vi "Manual Vi.vi"() -> ()   [LabVIEW 2015]
uses:
  IR/Control 1.ctl
  <vilib>/ni845x/ni845x.llb/ni845xControl.ctl
  <vilib>/MakerHub/LINX/Public/Peripherals/PWM/PWM Set Duty Cycle 1 Chan.vi
  <vilib>/MakerHub/LINX/Public/Peripherals/Digital/Digital Write 1 Chan.vi
  <vilib>/MakerHub/LINX/Public/Peripherals/Analog/Analog Read 1 Chan.vi
  <vilib>/MakerHub/LINX/Public/Peripherals/Analog/Analog Read N Chans.vi
  <vilib>/MakerHub/LINX/Public/Peripherals/Digital/Digital Write N Chans.vi
  <vilib>/MakerHub/LINX/Private/Local IO/LinxAnalogRead.vi
  <vilib>/MakerHub/LINX/Public/Utilities/Check Channel.vi
  <vilib>/MakerHub/LINX/Private/Local IO/LinxDigitalWrite.vi
  <vilib>/MakerHub/LINX/Public/Peripherals/PWM/PWM Set Duty Cycle N Chans.vi
  <vilib>/MakerHub/LINX/Private/Utilties/Generate Error.vi
  <vilib>/addons/control/pid/autopid.llb/PID Online Autotuning (Relay Feedback).vi
  <vilib>/addons/control/pid/pid.llb/PID Control Input Filter (DBL).vi
  <vilib>/addons/control/pid/NI_PID_pid.lvlib
  <vilib>/MakerHub/LINX/LMH-LINX.lvlib
  <vilib>/addons/control/pid/NI_PID_autopid.lvlib
  <instrlib>/Harvard Apparatus PHD Ultra Series/Harvard Apparatus PHD Ultra Series.lvlib
panel:
  out "LED already on? 5":bool
  out "LED already on? 4":bool
  out "LED already on? 3":bool
  out "LED already on? 2":bool
  out "LED already on? 1":bool
  in  "Flowrate":dbl=200.0
  in  "Pump Address":string="h"
  in  "LED On? 5":bool
  in  "LED On? 4":bool
  in  "LED On? 3":bool
  in  "LED On? 2":bool
  in  "LED On? 1":bool
  in  "HPLC with time(min)":dbl
  in  "Turn Valve and HPLC":bool
  in  "Turn HPLC":bool
  in  "Turn Valve":bool
  in  "Phase Sensor UB":dbl
  in  "Phase Sensor LB":dbl
  out "Pump On 7":bool=TRUE
  in  "Syringe Pump \n    Flowrate":dbl=200.0
  in  "Pump 7":bool
  out "Phase Sensor Chart":T1(graph)
  out "Phase_Sensor_voltage":dbl
  out "Temp SS 5":bool=TRUE
  out "Temp SS 4":bool=TRUE
  out "Temp SS 3":bool=TRUE
  out "Temp SS 2":bool=TRUE
  out "Temp SS 1":bool=TRUE
  in  "Temp On? 5":bool
  in  "Temp On? 4":bool
  in  "Temp On? 3":bool
  in  "Temp On? 2":bool
  in  "Temp On? 1":bool
  in  "Set Point 5":dbl
  in  "Set Point 4":dbl
  in  "Set Point 3":dbl
  in  "Set Point 2":dbl
  in  "Set Point 1":dbl
  in  "SSR Duration 5":dbl
  in  "SSR Duration 4":dbl
  in  "SSR Duration 3":dbl
  in  "SSR Duration 2":dbl
  in  "SSR Duration 1":dbl
  out "Pressure Chart 3":T1(graph)
  out "Flowrate Chart 3":T1(graph)
  out "System Error":bool=TRUE
  out "Flowrate Sensor 2":dbl format="%#_13g"
  out "Flowrate Sensor 1":dbl format="%#_13g"
  out "Pressure 2":dbl format="%#_13g"
  out "Pressure 1":dbl format="%#_13g"
  out "Error Message":string
  out "error out":errorcluster
  out "Temperature 4":dbl format="%#_g'C"
  out "Temperature 2":dbl format="%#_g'C"
  out "Temperature 5":dbl format="%#_g'C"
  out "Temperature 3":dbl format="%#_g'C"
  out "Temperature 1":dbl format="%#_g'C"
  out "Teperature Chart":T1(graph)
  out "Pump On 6":bool=TRUE
  out "Pump On 5":bool=TRUE
  out "Pump On 4":bool=TRUE
  out "Pump On 3":bool=TRUE
  out "Pump On 2":bool=TRUE
  out "Pump On 1":bool=TRUE
  in  "Stop Button":bool
  in  "Pump 6":bool
  in  "Pump 5":bool
  in  "Pump 4":bool
  in  "Pump 3":bool
  in  "Pump 2":bool
  in  "Pump 1":bool
  in  "Pump Address 6":string="h"
  in  "Pump Address 5":string="f"
  in  "Pump Address 4":string="e"
  in  "Pump Address 3":string="i"
  in  "Pump Address 2":string="j"
  in  "Pump Address 1":string="g"
  in  "Flowrate 6":dbl=200.0
  in  "Flowrate 5":dbl=200.0
  in  "Flowrate 4":dbl=200.0
  in  "Flowrate 3":dbl=200.0
  in  "Flowrate 2":dbl=200.0
  in  "Flowrate 1":dbl=200.0
  in  "COMM Port:: Harvard Syringe Pump":refnum<visa-resource-name>="COM5"
  in  "Sample Valve COMM::Port":refnum<visa-resource-name>="COM4"
  in  "IR Sensor Device":T2="USB0::0x3923::0x7514::01B3FF21::RAW"
  in  "Arduino COMM Port":refnum<visa-resource-name>="COM3"
  in  "COMM Port :: Milligat Pumps":T3="COM10"
  # "Molecules on Demand"
  # "Analytics"
  # "Pumps"
  # "Turn Valve and HPLC"
  # "Turn Valve"
  # "Turn on HPLC"
  # "Temperature Control"
  # "LED Reactors"
  # "Cooling Pump"
  # "Bay 2"
  # "Bay 3"
  # "Bay 1"
  # "Bay 4"
  # "Bay 5"
  # "Power On"
  # "Bay 1"
  # "Bay 2"
  # "Bay 3"
  # "Bay 4"
  # "Bay 5"
  # "Flowrates"
  # "Pressure"
  # "Temperature"
  # "Phase Sensor"
types:
  T1 = cluster{"[0]":dbl, "[1]":dbl, "[2]":dbl, "[3]":dbl, "[4]":dbl, "[5]":dbl, "[6]":dbl, "[7]":dbl, "[8]":dbl}
  T2 = typedef "ni845xControl.ctl" = refnum<k21>
  T3 = typedef "Control 1.ctl" = refnum<visa-resource-name>
  T4 = cluster{"Proportional gain Kc":dbl, "Integral time Ti (sec)":dbl, "Derivative time Ti (sec)":dbl}
  T5 = cluster{"type of controller":enum16{"P", "PI", "PID"}, "relay cycles":i32, "relay amplitude":dbl, "control specifications":enum16{"Fast", "Normal", "Slow"}, "PV noise level":dbl}
  T6 = typedef "LMH-LINX.lvlib/LINX Ref.ctl" = cluster{"IO":T7, "Interface":T8, "LINX Device Config":T9}
  T7 = typedef "LMH-LINX.lvlib/Platform.ctl" = enum16{"Remote", "Local"}
  T8 = typedef "LMH-LINX.lvlib/Interface.ctl" = enum16{"Serial", "TCP"}
  T9 = typedef "LMH-LINX.lvlib/Device.lvlib/LINX Device Config.ctl" = cluster{"Interface":T8, "COM Port":refnum<visa-resource-name>, "TCP Configuration":T10, "Device Family":u8, "Device ID":u8, "Device Name":string, "TCP Ref":refnum<k5>, "Channels":T11}
  T10 = typedef "LMH-LINX.lvlib/Device.lvlib/TCP Config.ctl" = cluster{"IP Address":string, "Port":u16}
  T11 = typedef "LMH-LINX.lvlib/Channels.ctl" = cluster{"DI":u8[], "DO":u8[], "AI":u8[], "AO":u8[], "PWM":u8[], "QE":u8[], "UART":u8[], "I2C 2":u8[], "SPI":u8[], "CAN":u8[], "Servo":u8[], "AI Ref (V)":dbl, "AI Resolution (Bits)":u8, "AO Ref (V)":dbl, "AO Resolution (Bits)":u8}
  T12 = cluster{"proportional gain (Kc)":dbl, "integral time (Ti, min)":dbl, "derivative time (Td, min)":dbl}
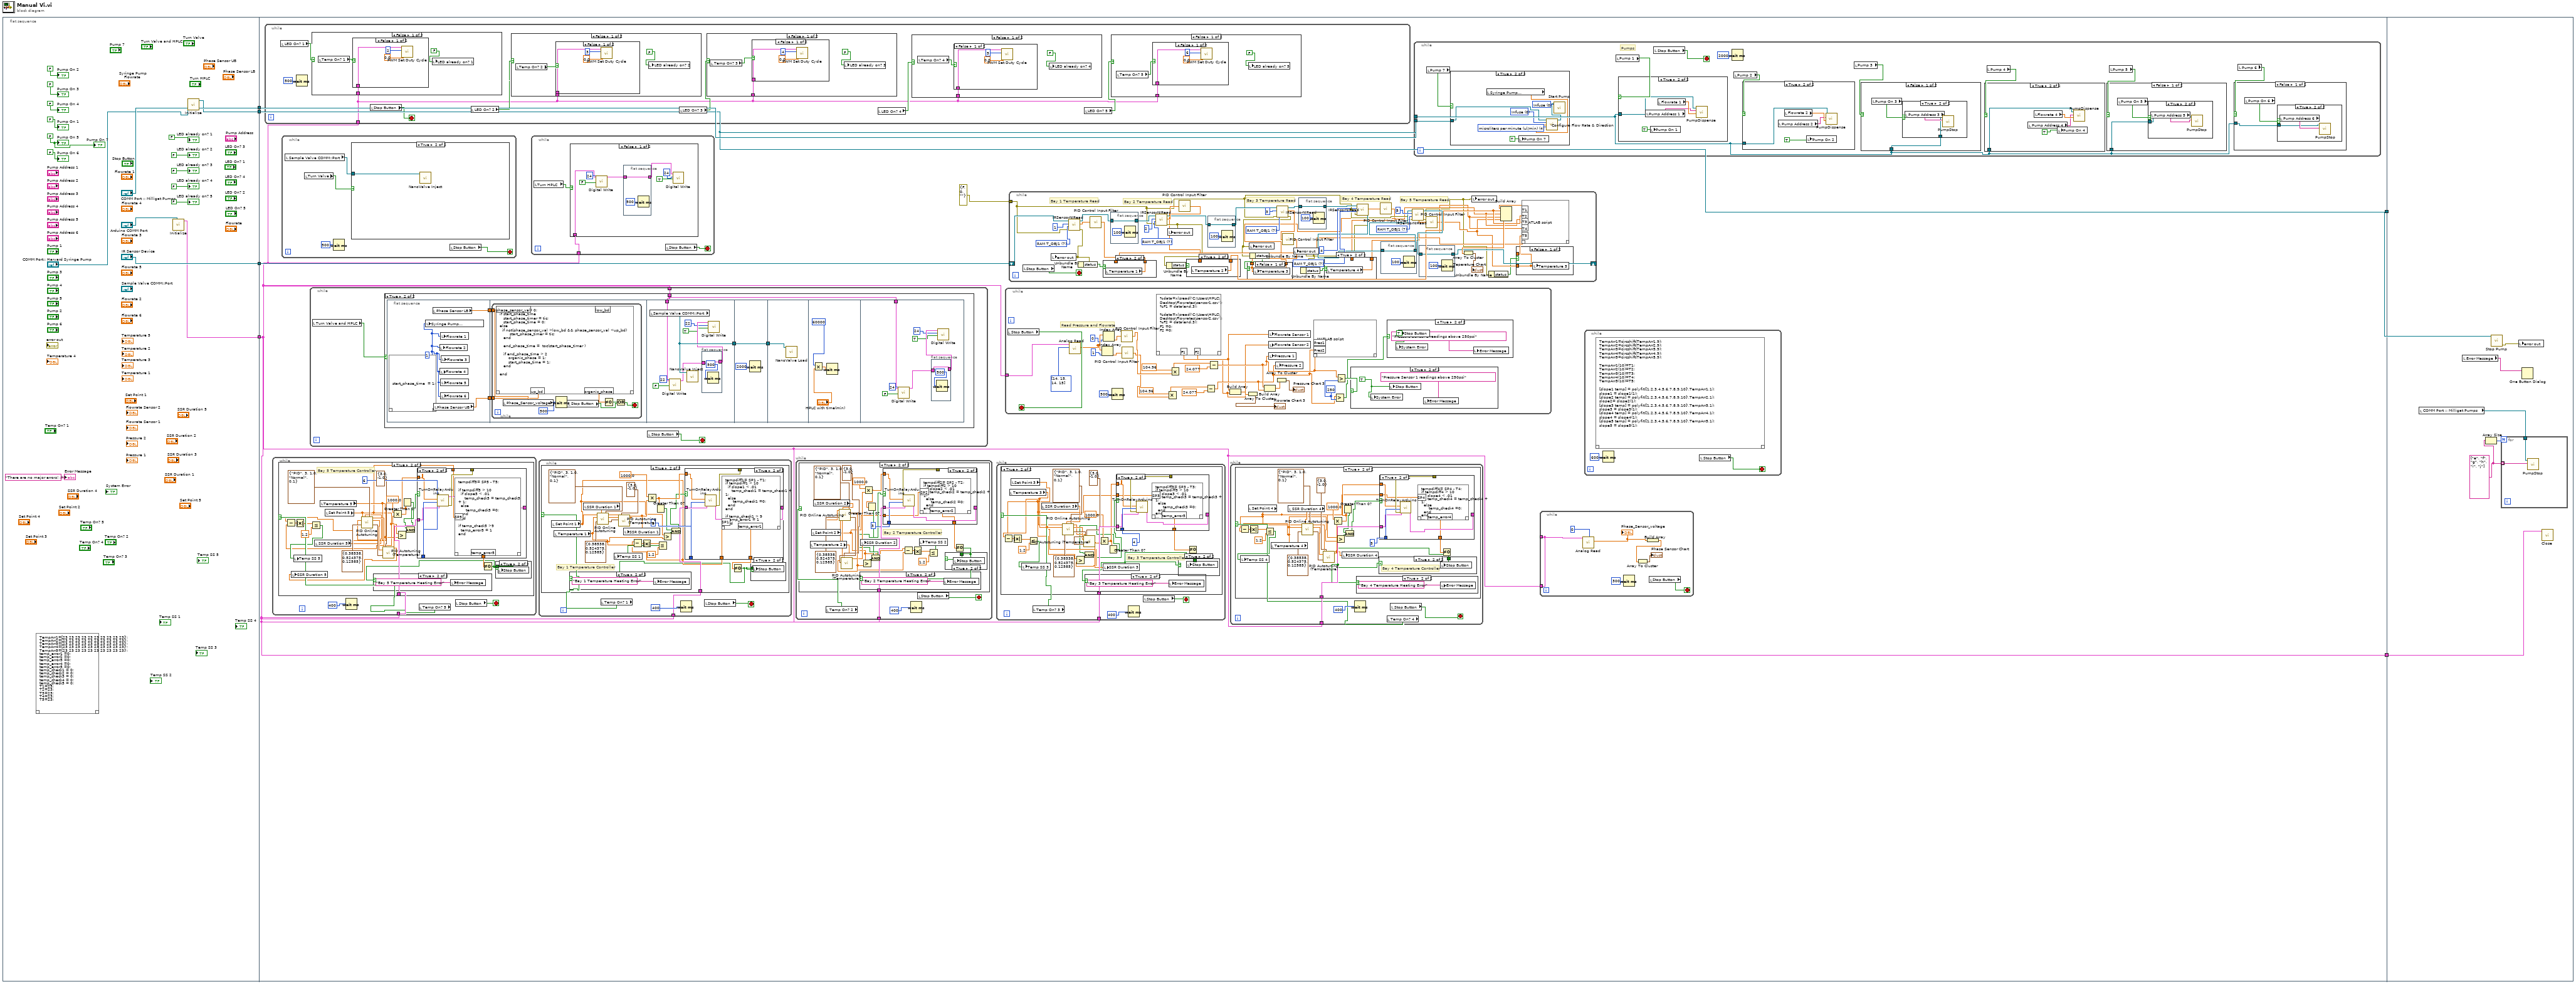
[diagram p0: block diagram]
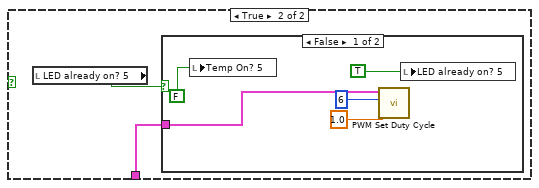
[diagram p3: hidden frame]
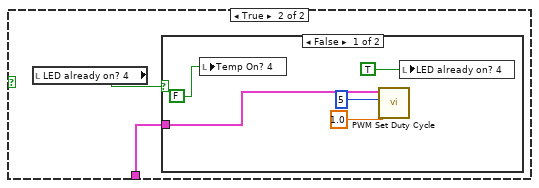
[diagram p6: hidden frame]
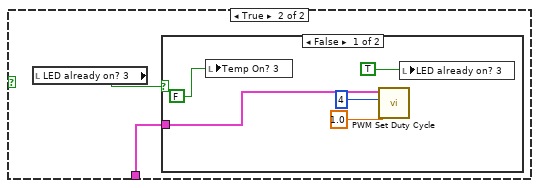
[diagram p9: hidden frame]
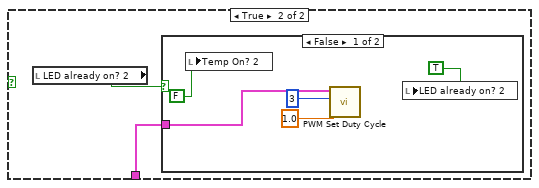
[diagram p12: hidden frame]
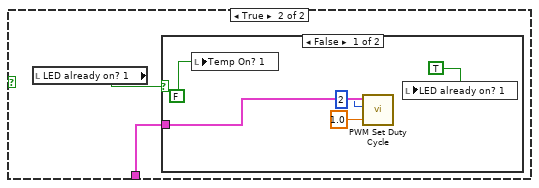
[diagram p15: hidden frame]
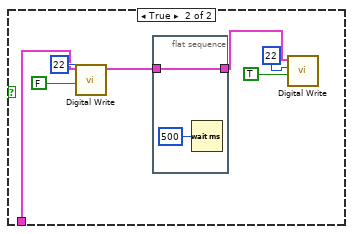
[diagram p18: hidden frame]
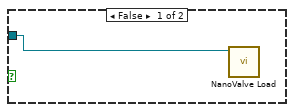
[diagram p19: hidden frame]
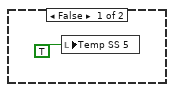
[diagram p20: hidden frame]
diagram:
  n1 = flat-sequence {
    tunnel: ["COMM Port :: Milligat Pumps"] -> w6
    tunnel: ["IR Sensor Device"] -> w5
    tunnel: [w16] -> w4
    tunnel: [w12] -> w2
    tunnel: w6 -> [w29]
    tunnel: w5 -> [w27]
    tunnel: w4 -> [w25]
    tunnel: [w25] -> w3
    tunnel: w2 -> [w26]
    tunnel: [w26] -> w1
    tunnel: w3 -> [w571]
    tunnel: w1 -> [w570]
    frame #0 {
      w14 = FALSE
      n2 = script code="TempArr1=[23 23 23 23 23 23 23 23 23 23]';\nTempArr2=[23 23 23 23 23 23 23 23 23 23]';\nTempArr3=[23 23 23 23 23 23 23 23 23 23]';\nTempArr4=[23 23 23 23 23 23 23 23 23 23]';\nTempArr5=[23 23 23 23 23 23 23 23 23 23]';\ntemp_error1 =0;\ntemp_error2 =0;\ntemp_error3 =0;\ntemp_error4 =0;\ntemp_error5 =0;\ntemp_check1 = 0;\ntemp_check2 = 0;\ntemp_check3 = 0;\ntemp_check4 = 0;\ntemp_check5 = 0;\nT1=23;\nT2=23;\nT3=23;\nT4=23;\nT5=23;"() -> ()  [unwired: 1 in, 1 out]
      n3 = call <instrlib>:"Initialize.vi"("Serial Port"="Arduino COMM Port") -> ("LINX Resource"=w16:T6)  [unwired: 8 in, 2 out]
      n4 = call <instrlib>:"Initialize.vi"("VISA resource name"="COMM Port:: Harvard Syringe Pump") -> ("VISA resource name out"=w12:refnum<visa-resource-name>)  [unwired: 9 in, 1 out]
      "Pump On 1" <- FALSE
      "Pump On 2" <- FALSE
      "Pump On 3" <- FALSE
      "Pump On 4" <- FALSE
      "Pump On 5" <- w14
      "Pump On 6" <- FALSE
      "Error Message" <- "There are no major errors! :)" ("Error Message")
      "Pump On 7" <- w14
      "LED already on? 1" <- FALSE ("LED already on? 1")
      "LED already on? 2" <- FALSE ("LED already on? 2")
      "LED already on? 3" <- FALSE ("LED already on? 3")
      "LED already on? 4" <- FALSE ("LED already on? 4")
      "LED already on? 5" <- FALSE ("LED already on? 5")
    }
    frame #1 {
      n5 = while {
        tunnel: w25 -> [w30]
        stop <- w37 stop-if-true
        n6 = local read "LED On? 1"() -> (w36:bool)
        n7 = Wait (ms)(milliseconds to wait=u32 500) -> ()  [unwired: 1 out]
        n8 = case shown="False" w36 {
          tunnel: w30 -> [w92 w96]
          frame False {
            n9 = local read "Temp On? 1"() -> (w90:bool)
            n10 = case shown="False" w90 {
              tunnel: w92 -> [w95 _]
              frame False {
                n11 = call-poly <vilib>:"PWM Set Duty Cycle.vi"("Duty Cycle (0-1)"=0.0, "PWM Channel"=u8 2, "LINX Resource"=w95) -> ()  [unwired: 7 in, 2 out]
              }
              frame True {
              }
            }
            n12 = local write "LED already on? 1"(FALSE ("LED already on? 2")) -> ()
          }
          frame True {
            n13 = local read "LED already on? 1"() -> (w97:bool)
            n14 = case shown="False" w97 {
              tunnel: w96 -> [w102 _]
              frame False {
                n15 = local write "Temp On? 1"(FALSE ("LED already on? 2")) -> ()
                n16 = call-poly <vilib>:"PWM Set Duty Cycle.vi"("Duty Cycle (0-1)"=1.0, "PWM Channel"=u8 2, "LINX Resource"=w102) -> ()  [unwired: 7 in, 2 out]
                n17 = local write "LED already on? 1"(TRUE ("LED already on? 2")) -> ()
              }
              frame True {
              }
            }
          }
        }
        n18 = local read "Stop Button"() -> (w37:bool)
        n19 = local read "LED On? 2"() -> (w34:bool)
        n20 = case shown="False" w34 {
          tunnel: w30 -> [w79 w83]
          frame False {
            n21 = local read "Temp On? 2"() -> (w77:bool)
            n22 = case shown="False" w77 {
              tunnel: w79 -> [w82 _]
              frame False {
                n23 = call-poly <vilib>:"PWM Set Duty Cycle.vi"("Duty Cycle (0-1)"=0.0, "PWM Channel"=u8 3, "LINX Resource"=w82) -> ()  [unwired: 7 in, 2 out]
              }
              frame True {
              }
            }
            n24 = local write "LED already on? 2"(FALSE ("LED already on? 2")) -> ()
          }
          frame True {
            n25 = local read "LED already on? 2"() -> (w84:bool)
            n26 = case shown="False" w84 {
              tunnel: w83 -> [w89 _]
              frame False {
                n27 = local write "Temp On? 2"(FALSE ("LED already on? 2")) -> ()
                n28 = call-poly <vilib>:"PWM Set Duty Cycle.vi"("Duty Cycle (0-1)"=1.0, "PWM Channel"=u8 3, "LINX Resource"=w89) -> ()  [unwired: 7 in, 2 out]
                n29 = local write "LED already on? 2"(TRUE ("LED already on? 2")) -> ()
              }
              frame True {
              }
            }
          }
        }
        n30 = local read "LED On? 3"() -> (w33:bool)
        n31 = case shown="False" w33 {
          tunnel: w30 -> [w66 w70]
          frame False {
            n32 = local read "Temp On? 3"() -> (w64:bool)
            n33 = case shown="False" w64 {
              tunnel: w66 -> [w69 _]
              frame False {
                n34 = call-poly <vilib>:"PWM Set Duty Cycle.vi"("Duty Cycle (0-1)"=0.0, "PWM Channel"=u8 4, "LINX Resource"=w69) -> ()  [unwired: 7 in, 2 out]
              }
              frame True {
              }
            }
            n35 = local write "LED already on? 3"(FALSE ("LED already on? 2")) -> ()
          }
          frame True {
            n36 = local read "LED already on? 3"() -> (w71:bool)
            n37 = case shown="False" w71 {
              tunnel: w70 -> [w76 _]
              frame False {
                n38 = local write "Temp On? 3"(FALSE ("LED already on? 2")) -> ()
                n39 = call-poly <vilib>:"PWM Set Duty Cycle.vi"("Duty Cycle (0-1)"=1.0, "PWM Channel"=u8 4, "LINX Resource"=w76) -> ()  [unwired: 7 in, 2 out]
                n40 = local write "LED already on? 3"(TRUE ("LED already on? 2")) -> ()
              }
              frame True {
              }
            }
          }
        }
        n41 = local read "LED On? 4"() -> (w32:bool)
        n42 = case shown="False" w32 {
          tunnel: w30 -> [w53 w57]
          frame False {
            n43 = local read "Temp On? 4"() -> (w51:bool)
            n44 = case shown="False" w51 {
              tunnel: w53 -> [w56 _]
              frame False {
                n45 = call-poly <vilib>:"PWM Set Duty Cycle.vi"("Duty Cycle (0-1)"=0.0, "PWM Channel"=u8 5, "LINX Resource"=w56) -> ()  [unwired: 7 in, 2 out]
              }
              frame True {
              }
            }
            n46 = local write "LED already on? 4"(FALSE ("LED already on? 2")) -> ()
          }
          frame True {
            n47 = local read "LED already on? 4"() -> (w58:bool)
            n48 = case shown="False" w58 {
              tunnel: w57 -> [w63 _]
              frame False {
                n49 = local write "Temp On? 4"(FALSE ("LED already on? 2")) -> ()
                n50 = call-poly <vilib>:"PWM Set Duty Cycle.vi"("Duty Cycle (0-1)"=1.0, "PWM Channel"=u8 5, "LINX Resource"=w63) -> ()  [unwired: 7 in, 2 out]
                n51 = local write "LED already on? 4"(TRUE ("LED already on? 2")) -> ()
              }
              frame True {
              }
            }
          }
        }
        n52 = local read "LED On? 5"() -> (w31:bool)
        n53 = case shown="False" w31 {
          tunnel: w30 -> [w40 w44]
          frame False {
            n54 = local read "Temp On? 5"() -> (w38:bool)
            n55 = case shown="False" w38 {
              tunnel: w40 -> [w43 _]
              frame False {
                n56 = call-poly <vilib>:"PWM Set Duty Cycle.vi"("Duty Cycle (0-1)"=0.0, "PWM Channel"=u8 6, "LINX Resource"=w43) -> ()  [unwired: 7 in, 2 out]
              }
              frame True {
              }
            }
            n57 = local write "LED already on? 5"(FALSE ("LED already on? 2")) -> ()
          }
          frame True {
            n58 = local read "LED already on? 5"() -> (w45:bool)
            n59 = case shown="False" w45 {
              tunnel: w44 -> [w50 _]
              frame False {
                n60 = local write "Temp On? 5"(FALSE ("LED already on? 2")) -> ()
                n61 = call-poly <vilib>:"PWM Set Duty Cycle.vi"("Duty Cycle (0-1)"=1.0, "PWM Channel"=u8 6, "LINX Resource"=w50) -> ()  [unwired: 7 in, 2 out]
                n62 = local write "LED already on? 5"(TRUE ("LED already on? 2")) -> ()
              }
              frame True {
              }
            }
          }
        }
      }
      n63 = while {
        tunnel: w25 -> [w187]
        stop <- w186 stop-if-true
        n64 = Wait (ms)(milliseconds to wait=u32 400) -> ()  [unwired: 1 out]
        n65 = local read "Temp On? 5"() -> (w185:bool)
        n66 = case shown="True" w185 {
          tunnel: w187 -> [_ w211]
          frame False {
            n67 = local write "Temp SS 5"(TRUE ("Temp SS? 5")) -> ()
          }
          frame True {
            # "Bay 5 Temperature Controller"
            n68 = local read "SSR Duration 5"() -> (w201:dbl)
            n69 = local read "Temperature 5"() -> (w193:dbl)
            n70 = local read "Set Point 5"() -> (w191:dbl)
            n71 = Subtract(x=w193, y=w191) -> (x-y=w198:dbl)
            n72 = Absolute Value(x=w198) -> (abs(x)=w200:dbl)
            n73 = Less Or Equal?(x=w200, y=1.2) -> (x <= y?=w197:bool)
            n74 = local write "Temp SS 5"(w197) -> ()
            n75 = call-poly <vilib>:"PID Online Autotuning.vi"("setpoint"=w191, "manipulated variable"=w201, "autotuning parameters"=T5 {"type of controller"=enum."PID", "relay cycles"=3, "relay amplitude"=1.0, "control specifications"=enum."Normal", "PV noise level"=0.1} ("Autotuning Parameters R1"), "process variable"=w193, "PID gains in"=T4 {"Proportional gain Kc"=0.38538, "Integral time Ti (sec)"=0.524375, "Derivative time Ti (sec)"=0.12585} ("PID gains 2")) -> ("setpoint out"=w203:dbl, "process variable out"=w204:dbl, "PID gains out"=w206:T12)  [unwired: 6 in, 2 out]
            n76 = call <vilib>:"PID Autotuning (Temperature).vi"("desired temperature"=w203, "measured temperature"=w204, "PID gains in"=w206, "output range"=cluster{"output high":dbl, "output low":dbl} {"output high"=3.0, "output low"=-1.0} ("Output range")) -> ("output"=w202:dbl)  [unwired: 12 in, 3 out]
            n77 = local write "SSR Duration 5"(w202) -> ()
            n78 = Multiply(x=1000.0, y=w202) -> (x*y=w210:dbl)
            n79 = Greater?(x=w191, y=w193) -> (0:w194:bool)
            n80 = Greater Than 0?(x=w210) -> (x > 0?=w196:bool)
            n81 = And(x=w196, y=w194) -> (x .and. y?=w195:bool)
            n82 = case shown="True" w195 {
              tunnel: [errorcluster {"status"=FALSE, "code"=0, "source"=""} ("error out") w225] -> _
              tunnel: 6 -> [_ w226]
              tunnel: [w217 w224] -> _
              tunnel: w211 -> [w217 w223]
              tunnel: w210 -> [w216 w222]
              tunnel: [0.0 w221] -> w192
              tunnel: w191 -> [_ w220]
              frame False {
                n83 = Absolute Value(x=w216) -> (abs(x)=w218:dbl)
                n84 = Wait (ms)(milliseconds to wait=w218) -> ()  [unwired: 1 out]
              }
              frame True {
                n85 = call "TurnOnRelayArduino.vi"("channel"=w226, "duration"=w222, "LINX Resource"=w223) -> ("error out"=w225:errorcluster, "LINX Resource Out"=w224:T6)  [unwired: 7 in]
                n86 = script code="tempdiff5= SP5 - T5;\n\nif tempdiff5 > 10\n  if slope5 < .01\n     temp_check5 = temp_check5 + 1;\n  else\n      temp_check5 =0;\n  end\nend\n\nif temp_check5 >9\n  temp_error5 = 1\nend"("SP5"=w220) -> ("temp_error5"=w221:dbl)  [unwired: 1 in, 1 out]
              }
            }
            n87 = Not Equal To 0?(x=w192) -> (x != 0?=w190:bool)
            n88 = case shown="True" w190 {
              frame False {
              }
              frame True {
                n89 = local write "Error Message"("Bay 5 Temperature Heating Error") -> ()
              }
            }
            n90 = case shown="True" w190 {
              tunnel: w190 -> [_ w213]
              frame False {
              }
              frame True {
                n91 = local write "Stop Button"(w213) -> ()
              }
            }
          }
        }
        n92 = local read "Stop Button"() -> (w186:bool)
      }
      n93 = while {
        stop <- w175 stop-if-true
        n94 = local read "Sample Valve COMM::Port"() -> (w172:refnum<visa-resource-name>)
        n95 = local read "Turn Valve"() -> (w173:bool)
        n96 = Wait (ms)(milliseconds to wait=u32 500) -> ()  [unwired: 1 out]
        n97 = case shown="True" w173 {
          tunnel: w172 -> [w176 w177]
          frame False {
            n98 = call "NanoValve Load.vi"("VISA resource name"=w176) -> ()  [unwired: 10 in, 1 out]
          }
          frame True {
            n99 = call "NanoValve Inject.vi"("VISA resource name"=w177) -> ()  [unwired: 10 in, 1 out]
          }
        }
        n100 = local read "Stop Button"() -> (w175:bool)
      }
      n101 = while {
        tunnel: w25 -> [w105]
        stop <- w107 stop-if-true
        n102 = local read "Turn Valve and HPLC"() -> (w106:bool)
        n103 = case shown="True" w106 {
          tunnel: w105 -> [_ w108]
          frame False {
          }
          frame True {
            n104 = flat-sequence {
              tunnel: [w114] -> w110
              tunnel: [w113] -> w109
              tunnel: w110 -> [w117]
              tunnel: w109 -> [w116]
              tunnel: w108 -> [w131]
              tunnel: [w130] -> w111
              tunnel: [w136] -> w112
              tunnel: w111 -> [w136]
              tunnel: w112 -> [w138]
              tunnel: w108 -> [w142]
              frame #0 {
                w115 = 1
                n105 = script code="start_phase_time  = 1;"() -> ()  [unwired: 1 in, 1 out]
                n106 = local write "Syringe Pump \n    Flowrate"(w115) -> ()
                n107 = local read "Phase Sensor LB"() -> (w113:dbl)
                n108 = local read "Phase Sensor UB"() -> (w114:dbl)
                n109 = local write "Flowrate 2"(w115) -> ()
                n110 = local write "Flowrate 4"(w115) -> ()
                n111 = local write "Flowrate 1"(w115) -> ()
                n112 = local write "Flowrate 5"(w115) -> ()
                n113 = local write "Flowrate 6"(w115) -> ()
                n114 = local write "Flowrate 3"(w115) -> ()
              }
              frame #1 {
                n115 = while {
                  tunnel: w117 -> [w119]
                  tunnel: w116 -> [w118]
                  stop <- w122 stop-if-true
                  n116 = local read "Phase_Sensor_voltage"() -> (w125:dbl)
                  n117 = script code="organic_phase = 0;\nif start_phase_time \n   start_phase_timer = tic;\n   start_phase_time = 0;\nelse\n  if not(phase_sensor_val >low_bd && phase_sensor_val <up_bd)\n        start_phase_timer = tic;\n   end\n\n   end_phase_time =  toc(start_phase_timer )\n\n   if end_phase_time > 2\n       organic_phase = 1;\n       start_phase_time = 1;\n   end\n\nend"("phase_sensor_val"=w125, "low_bd"=w118, "up_bd"=w119) -> ("organic_phase"=w124:dbl)  [unwired: 1 in, 1 out]
                  n118 = Wait (ms)(milliseconds to wait=500) -> ()  [unwired: 1 out]
                  n119 = local read "Stop Button"() -> (w121:bool)
                  n120 = Not Equal To 0?(x=w124) -> (x != 0?=w123:bool)
                  n121 = Or(x=w123, y=w121) -> (x .or. y?=w122:bool)
                }
              }
              frame #2 {
                n122 = local read "Sample Valve COMM::Port"() -> (w130:refnum<visa-resource-name>)
                n123 = call-poly <vilib>:"Digital Write.vi"("Output Value"=FALSE, "DO Channel"=u8 22, "LINX Resource"=w131) -> ("LINX Resource"=w129:T6)  [unwired: 7 in, 1 out]
                n124 = call "NanoValve Inject.vi"("VISA resource name"=w130) -> ()  [unwired: 10 in, 1 out]
                n125 = flat-sequence {
                  tunnel: [w134] -> _
                  tunnel: w129 -> [w134]
                  tunnel: [w134] -> w128
                  frame #0 {
                    n126 = Wait (ms)(milliseconds to wait=u32 500) -> ()  [unwired: 1 out]
                  }
                }
                n127 = call-poly <vilib>:"Digital Write.vi"("Output Value"=TRUE, "DO Channel"=u8 22, "LINX Resource"=w128) -> ()  [unwired: 7 in, 2 out]
              }
              frame #3 {
                n128 = Wait (ms)(milliseconds to wait=u32 2000) -> ()  [unwired: 1 out]
              }
              frame #4 {
                n129 = call "NanoValve Load.vi"("VISA resource name"=w138) -> ()  [unwired: 10 in, 1 out]
              }
              frame #5 {
                n130 = Multiply(x=u32 60000 ("milliseconds to wait"), y="HPLC with time(min)") -> (x*y=w140:dbl)
                n131 = Wait (ms)(milliseconds to wait=w140) -> ()  [unwired: 1 out]
              }
              frame #6 {
                n132 = call-poly <vilib>:"Digital Write.vi"("Output Value"=FALSE, "DO Channel"=u8 24, "LINX Resource"=w142) -> ("LINX Resource"=w146:T6)  [unwired: 7 in, 1 out]
                n133 = flat-sequence {
                  tunnel: w146 -> [w149]
                  tunnel: [w149] -> w145
                  frame #0 {
                    n134 = Wait (ms)(milliseconds to wait=u32 500) -> ()  [unwired: 1 out]
                  }
                }
                n135 = call-poly <vilib>:"Digital Write.vi"("Output Value"=TRUE, "DO Channel"=u8 24, "LINX Resource"=w145) -> ()  [unwired: 7 in, 2 out]
              }
            }
          }
        }
        n136 = local read "Stop Button"() -> (w107:bool)
      }
      n137 = while {
        tunnel: w25 -> [w151]
        stop <- w153 stop-if-true
        n138 = local read "Turn HPLC"() -> (w152:bool)
        n139 = case shown="False" w152 {
          tunnel: w151 -> [w154 w167]
          frame False {
            n140 = call-poly <vilib>:"Digital Write.vi"("Output Value"=FALSE, "DO Channel"=u8 24, "LINX Resource"=w154) -> ("LINX Resource"=w158:T6)  [unwired: 7 in, 1 out]
            n141 = flat-sequence {
              tunnel: [w161] -> w155
              tunnel: w158 -> [w161]
              frame #0 {
                n142 = Wait (ms)(milliseconds to wait=u32 500) -> ()  [unwired: 1 out]
              }
            }
            n143 = call-poly <vilib>:"Digital Write.vi"("Output Value"=TRUE, "DO Channel"=u8 24, "LINX Resource"=w155) -> ()  [unwired: 7 in, 2 out]
          }
          frame True {
            n144 = call-poly <vilib>:"Digital Write.vi"("Output Value"=FALSE, "DO Channel"=u8 22, "LINX Resource"=w167) -> ("LINX Resource"=w166:T6)  [unwired: 7 in, 1 out]
            n145 = flat-sequence {
              tunnel: [w170] -> w163
              tunnel: w166 -> [w170]
              frame #0 {
                n146 = Wait (ms)(milliseconds to wait=u32 500) -> ()  [unwired: 1 out]
              }
            }
            n147 = call-poly <vilib>:"Digital Write.vi"("Output Value"=TRUE, "DO Channel"=u8 22, "LINX Resource"=w163) -> ()  [unwired: 7 in, 2 out]
          }
        }
        n148 = local read "Stop Button"() -> (w153:bool)
      }
      n149 = while {
        tunnel: w25 -> [w354]
        stop <- w356 stop-if-true
        n150 = local read "Temp On? 1"() -> (w353:bool)
        n151 = case shown="True" w353 {
          tunnel: w354 -> [_ w370]
          frame False {
            n152 = local write "Temp SS 1"(TRUE ("Temp SS? 1")) -> ()
          }
          frame True {
            # "Bay 1 Temperature Controller"
            n153 = local read "Set Point 1"() -> (w359:dbl)
            n154 = local read "Temperature 1"() -> (w361:dbl)
            n155 = local read "SSR Duration 1"() -> (w374:dbl)
            n156 = call-poly <vilib>:"PID Online Autotuning.vi"("setpoint"=w359, "manipulated variable"=w374, "autotuning parameters"=T5 {"type of controller"=enum."PID", "relay cycles"=3, "relay amplitude"=1.0, "control specifications"=enum."Normal", "PV noise level"=0.1} ("Autotuning Parameters R1"), "process variable"=w361, "PID gains in"=T4 {"Proportional gain Kc"=0.38538, "Integral time Ti (sec)"=0.524375, "Derivative time Ti (sec)"=0.12585} ("PID gains 2")) -> ("setpoint out"=w380:dbl, "process variable out"=w379:dbl, "PID gains out"=w376:T12)  [unwired: 6 in, 2 out]
            n157 = call <vilib>:"PID Autotuning (Temperature).vi"("desired temperature"=w380, "measured temperature"=w379, "plant parameters in"=w376, "output range"=cluster{"output high":dbl, "output low":dbl} {"output high"=3.0, "output low"=-1.0} ("Output range")) -> ("output"=w372:dbl)  [unwired: 12 in, 3 out]
            n158 = local write "SSR Duration 1"(w372) -> ()
            n159 = Subtract(x=w359, y=w361) -> (x-y=w365:dbl)
            n160 = Absolute Value(x=w365) -> (abs(x)=w368:dbl)
            n161 = Multiply(x=1000.0, y=w372) -> (x*y=w369:dbl)
            n162 = Greater Than 0?(x=w369) -> (x > 0?=w362:bool)
            n163 = Less Or Equal?(x=w368, y=1.2) -> (x <= y?=w366:bool)
            n164 = local write "Temp SS 1"(w366) -> ()
            n165 = Greater?(x=w359, y=w361) -> (0:w364:bool)
            n166 = And(x=w362, y=w364) -> (x .and. y?=w363:bool)
            n167 = case shown="True" w363 {
              tunnel: [errorcluster {"status"=FALSE, "code"=0, "source"=""} ("error out") w392] -> _
              tunnel: w370 -> [w385 w394]
              tunnel: 2 -> [_ w393]
              tunnel: [w385 w391] -> _
              tunnel: w369 -> [w384 w390]
              tunnel: [0.0 w389] -> w360
              tunnel: w359 -> [_ w388]
              frame False {
                n168 = Absolute Value(x=w384) -> (abs(x)=w386:dbl)
                n169 = Wait (ms)(milliseconds to wait=w386) -> ()  [unwired: 1 out]
              }
              frame True {
                n170 = call "TurnOnRelayArduino.vi"("channel"=w393, "duration"=w390, "LINX Resource"=w394) -> ("error out"=w392:errorcluster, "LINX Resource Out"=w391:T6)  [unwired: 7 in]
                n171 = script code="tempdiff1= SP1 - T1;\nif tempdiff1 > 10\n  if slope1 < .01\n     temp_check1 = temp_check1 + 1;\n  else\n      temp_check1 =0;\n  end\nend\n\nif temp_check1 > 9\n  temp_error1 = 1\nend"("SP1"=w388) -> ("temp_error1"=w389:dbl)  [unwired: 1 in, 1 out]
              }
            }
            n172 = Not Equal To 0?(x=w360) -> (x != 0?=w358:bool)
            n173 = case shown="True" w358 {
              frame False {
              }
              frame True {
                n174 = local write "Error Message"("Bay 1 Temperature Heating Error") -> ()
              }
            }
            n175 = case shown="True" w358 {
              tunnel: w358 -> [_ w381]
              frame False {
              }
              frame True {
                n176 = local write "Stop Button"(w381) -> ()
              }
            }
          }
        }
        n177 = Wait (ms)(milliseconds to wait=u32 400) -> ()  [unwired: 1 out]
        n178 = local read "Stop Button"() -> (w356:bool)
      }
      n179 = while {
        tunnel: w25 -> [w312]
        stop <- w314 stop-if-true
        n180 = local read "Temp On? 2"() -> (w311:bool)
        n181 = case shown="True" w311 {
          tunnel: w312 -> [_ w331]
          frame False {
            n182 = local write "Temp SS 2"(TRUE ("Temp SS? 2")) -> ()
          }
          frame True {
            # "Bay 2 Temperature Controller"
            n183 = local read "Temperature 2"() -> (w319:dbl)
            n184 = local read "Set Point 2"() -> (w317:dbl)
            n185 = local read "SSR Duration 2"() -> (w335:dbl)
            n186 = call-poly <vilib>:"PID Online Autotuning.vi"("setpoint"=w317, "manipulated variable"=w335, "autotuning parameters"=T5 {"type of controller"=enum."PID", "relay cycles"=3, "relay amplitude"=1.0, "control specifications"=enum."Normal", "PV noise level"=0.1} ("Autotuning Parameters R1"), "process variable"=w319, "PID gains in"=T4 {"Proportional gain Kc"=0.38538, "Integral time Ti (sec)"=0.524375, "Derivative time Ti (sec)"=0.12585} ("PID gains 2")) -> ("setpoint out"=w333:dbl, "process variable out"=w332:dbl, "PID gains out"=w338:T12)  [unwired: 6 in, 2 out]
            n187 = call <vilib>:"PID Autotuning (Temperature).vi"("desired temperature"=w333, "measured temperature"=w332, "plant parameters in"=w338, "output range"=cluster{"output high":dbl, "output low":dbl} {"output high"=3.0, "output low"=-1.0} ("Output range")) -> ("output"=w327:dbl)  [unwired: 12 in, 3 out]
            n188 = local write "SSR Duration 2"(w327) -> ()
            n189 = Greater?(x=w317, y=w319) -> (0:w322:bool)
            n190 = Multiply(x=1000.0, y=w327) -> (x*y=w329:dbl)
            n191 = Greater Than 0?(x=w329) -> (x > 0?=w320:bool)
            n192 = And(x=w320, y=w322) -> (x .and. y?=w321:bool)
            n193 = case shown="True" w321 {
              tunnel: [errorcluster {"status"=FALSE, "code"=0, "source"=""} ("error out") w350] -> _
              tunnel: w331 -> [w343 w352]
              tunnel: 3 -> [_ w351]
              tunnel: [w343 w349] -> _
              tunnel: w329 -> [w342 w348]
              tunnel: [0.0 w347] -> w318
              tunnel: w317 -> [_ w346]
              frame False {
                n194 = Absolute Value(x=w342) -> (abs(x)=w344:dbl)
                n195 = Wait (ms)(milliseconds to wait=w344) -> ()  [unwired: 1 out]
              }
              frame True {
                n196 = call "TurnOnRelayArduino.vi"("channel"=w351, "duration"=w348, "LINX Resource"=w352) -> ("error out"=w350:errorcluster, "LINX Resource Out"=w349:T6)  [unwired: 7 in]
                n197 = script code="tempdiff2= SP2 - T2;\nif tempdiff2 > 10\n  if slope2 < .01\n     temp_check2 = temp_check2 + 1;\n  else\n      temp_check2 =0;\n  end\nend\n\nif temp_check2 > 9\n  temp_error2 = 1\nend"("SP2"=w346) -> ("temp_error2"=w347:dbl)  [unwired: 1 in, 1 out]
              }
            }
            n198 = Subtract(x=w317, y=w319) -> (x-y=w324:dbl)
            n199 = Absolute Value(x=w324) -> (abs(x)=w326:dbl)
            n200 = Less Or Equal?(x=w326, y=1.2) -> (x <= y?=w323:bool)
            n201 = local write "Temp SS 2"(w323) -> ()
            n202 = Not Equal To 0?(x=w318) -> (x != 0?=w316:bool)
            n203 = case shown="True" w316 {
              frame False {
              }
              frame True {
                n204 = local write "Error Message"("Bay 2 Temperature Heating Error") -> ()
              }
            }
            n205 = case shown="True" w316 {
              tunnel: w316 -> [_ w339]
              frame False {
              }
              frame True {
                n206 = local write "Stop Button"(w339) -> ()
              }
            }
          }
        }
        n207 = Wait (ms)(milliseconds to wait=u32 400) -> ()  [unwired: 1 out]
        n208 = local read "Stop Button"() -> (w314:bool)
      }
      n209 = while {
        tunnel: w25 -> [w270]
        stop <- w271 stop-if-true
        n210 = local read "Temp On? 3"() -> (w269:bool)
        n211 = case shown="True" w269 {
          tunnel: w270 -> [_ w296]
          frame False {
            n212 = local write "Temp SS 3"(TRUE) -> ()
          }
          frame True {
            # "Bay 3 Temperature Controller"
            n213 = local read "Temperature 3"() -> (w279:dbl)
            n214 = local read "Set Point 3"() -> (w275:dbl)
            n215 = Subtract(x=w279, y=w275) -> (x-y=w282:dbl)
            n216 = Absolute Value(x=w282) -> (abs(x)=w284:dbl)
            n217 = Less Or Equal?(x=w284, y=1.2) -> (x <= y?=w281:bool)
            n218 = local write "Temp SS 3"(w281) -> ()
            n219 = local read "SSR Duration 3"() -> (w291:dbl)
            n220 = call-poly <vilib>:"PID Online Autotuning.vi"("setpoint"=w275, "manipulated variable"=w291, "autotuning parameters"=T5 {"type of controller"=enum."PID", "relay cycles"=3, "relay amplitude"=1.0, "control specifications"=enum."Normal", "PV noise level"=0.1} ("Autotuning Parameters R1"), "process variable"=w279, "PID gains in"=T4 {"Proportional gain Kc"=0.38538, "Integral time Ti (sec)"=0.524375, "Derivative time Ti (sec)"=0.12585} ("PID gains 2")) -> ("setpoint out"=w289:dbl, "process variable out"=w290:dbl, "PID gains out"=w293:T12)  [unwired: 6 in, 2 out]
            n221 = Greater?(x=w275, y=w279) -> (0:w280:bool)
            n222 = call <vilib>:"PID Autotuning (Temperature).vi"("desired temperature"=w289, "measured temperature"=w290, "PID gains in"=w293, "output range"=cluster{"output high":dbl, "output low":dbl} {"output high"=3.0, "output low"=-1.0} ("Output range")) -> ("output"=w286:dbl)  [unwired: 12 in, 3 out]
            n223 = Multiply(x=1000.0, y=w286) -> (x*y=w288:dbl)
            n224 = local write "SSR Duration 3"(w286) -> ()
            n225 = Greater Than 0?(x=w288) -> (x > 0?=w278:bool)
            n226 = And(x=w278, y=w280) -> (x .and. y?=w277:bool)
            n227 = case shown="True" w277 {
              tunnel: [errorcluster {"status"=FALSE, "code"=0, "source"=""} ("error out") w309] -> _
              tunnel: 4 -> [_ w310]
              tunnel: [w301 w308] -> _
              tunnel: w296 -> [w301 w307]
              tunnel: w288 -> [w300 w306]
              tunnel: [0.0 w305] -> w276
              tunnel: w275 -> [_ w304]
              frame False {
                n228 = Absolute Value(x=w300) -> (abs(x)=w302:dbl)
                n229 = Wait (ms)(milliseconds to wait=w302) -> ()  [unwired: 1 out]
              }
              frame True {
                n230 = call "TurnOnRelayArduino.vi"("channel"=w310, "duration"=w306, "LINX Resource"=w307) -> ("error out"=w309:errorcluster, "LINX Resource Out"=w308:T6)  [unwired: 7 in]
                n231 = script code="tempdiff3= SP3 - T3;\nif tempdiff3 > 10\n  if slope3 < .01\n     temp_check3 = temp_check3 + 1;\n  else\n      temp_check3 =0;\n  end\nend\n\nif temp_check3 > 9\n  temp_error3 = 1\nend"("SP3"=w304) -> ("temp_error3"=w305:dbl)  [unwired: 1 in, 1 out]
              }
            }
            n232 = Not Equal To 0?(x=w276) -> (x != 0?=w274:bool)
            n233 = case shown="True" w274 {
              frame False {
              }
              frame True {
                n234 = local write "Error Message"("Bay 3 Temperature Heating Error") -> ()
              }
            }
            n235 = case shown="True" w274 {
              tunnel: w274 -> [_ w297]
              frame False {
              }
              frame True {
                n236 = local write "Stop Button"(w297) -> ()
              }
            }
          }
        }
        n237 = Wait (ms)(milliseconds to wait=u32 400) -> ()  [unwired: 1 out]
        n238 = local read "Stop Button"() -> (w271:bool)
      }
      n239 = while {
        tunnel: w25 -> [w399]
        stop <- w422 stop-if-true
        w404 = 250
        # "Read Pressure and Flowrate"
        n240 = local read "Stop Button"() -> (w422:bool)
        n241 = call-poly <vilib>:"Analog Read.vi"("AI Channel(s)"=i32[] [14, 15, 14, 15], "LINX Resource"=w399) -> ("Voltages"=w420:dbl[])  [unwired: 6 in, 3 out]
        n242 = Index Array(array=w420, index=1) -> (element=w416:dbl)
        n243 = Index Array(array=w420, index=0) -> (element=w417:dbl)
        n244 = Wait (ms)(milliseconds to wait=u32 500) -> ()  [unwired: 1 out]
        n245 = call-poly <vilib>:"PID Control Input Filter.vi"("input"=w417) -> ("output"=w398:dbl)  [unwired: 4 in]
        n246 = call-poly <vilib>:"PID Control Input Filter.vi"("input"=w416) -> ("output"=w397:dbl)  [unwired: 4 in]
        n247 = script code="%data=xlsread('C:\\Users\\HPLC\\Desktop\\Flowrates\\sensor1.csv');\n%F1 = data(end,3);\n\n%data=xlsread('C:\\Users\\HPLC\\Desktop\\Flowrates\\sensor2.csv');\n%F2 = data(end,3);\nF1 =0;\nF2 =0;"() -> ("F1"=w396:dbl, "F2"=w395:dbl)  [unwired: 1 in, 1 out]
        n248 = Multiply(x=104.96 ("y"), y=w397) -> (x*y=w410:dbl)
        n249 = Multiply(x=104.96 ("y"), y=w398) -> (x*y=w413:dbl)
        n250 = Subtract(x=w410, y=24.077) -> (x-y=w402:dbl)
        n251 = Subtract(x=w413, y=24.077) -> (x-y=w403:dbl)
        n252 = Build Array(w396, w395) -> (w407:dbl[])
        n253 = Array To Cluster(array=w407) -> (cluster=→"Flowrate Chart 3":T1)
        n254 = Build Array(w403, w402) -> (w408:dbl[])
        n255 = local write "Flowrate Sensor 1"(w396) -> ()
        n256 = local write "Flowrate Sensor 2"(w395) -> ()
        n257 = local write "Pressure 1"(w403) -> ()
        n258 = local write "Pressure 2"(w402) -> ()
        n259 = Array To Cluster(array=w408) -> (cluster=→"Pressure Chart 3":T1)
        n260 = script code="MATLAB script"("Pres1"=w403, "Pres2"=w402) -> ()  [unwired: 1 in, 1 out]
        n261 = Greater?(x=w402, y=w404) -> (0:w400:bool)
        n262 = Greater?(x=w403, y=w404) -> (0:w401:bool)
        n263 = case shown="True" w401 {
          frame False {
          }
          frame True {
            w426 = TRUE ("Stop")
            n264 = local write "System Error"(w426) -> ()
            n265 = local write "Stop Button"(w426) -> ()
            n266 = local write "Error Message"("Pressure Sensor 1 readings above 250psi") -> ()
          }
        }
        n267 = case shown="True" w400 {
          frame False {
          }
          frame True {
            w424 = TRUE ("Stop")
            n268 = local write "System Error"(w424) -> ()
            n269 = local write "Stop Button"(w424) -> ()
            n270 = local write "Error Message"("Pressure Sensor 2 readings above 250psi") -> ()
          }
        }
      }
      n271 = while {
        shift-right: [w448] -> _
        shift-left: w27 -> [w449]
        tunnel: errorcluster {"status"=FALSE, "code"=0, "source"=""} ("error out") -> [w447]
        stop <- w473 stop-if-true
        w464 = u8 7 items=["RAM IR raw  Ch1"=4, "RAM IR raw  Ch2"=5, "RAM T_A"=6, "RAM T_OBJ1"=7, "RAM T_OBJ2"=8, "EEPROM_To_max"=32, "EEPROM_To_min"=33, "EEPROM_PWM_CTRL"=34, "EEPROM_Ta_range"=35, "EEPROM_Emissivity_CorrCoeff"=36, "EEPROM_SMBus Address"=46, "EEPROM_ConfigReg"=37] ("Melexis_Cmmds")
        w466 = u8 7 items=["RAM IR raw  Ch1"=4, "RAM IR raw  Ch2"=5, "RAM T_A"=6, "RAM T_OBJ1"=7, "RAM T_OBJ2"=8, "EEPROM_To_max"=32, "EEPROM_To_min"=33, "EEPROM_PWM_CTRL"=34, "EEPROM_Ta_range"=35, "EEPROM_Emissivity_CorrCoeff"=36, "EEPROM_SMBus Address"=46, "EEPROM_ConfigReg"=37] ("Melexis_Cmmds")
        w465 = u8 7 items=["RAM IR raw  Ch1"=4, "RAM IR raw  Ch2"=5, "RAM T_A"=6, "RAM T_OBJ1"=7, "RAM T_OBJ2"=8, "EEPROM_To_max"=32, "EEPROM_To_min"=33, "EEPROM_PWM_CTRL"=34, "EEPROM_Ta_range"=35, "EEPROM_Emissivity_CorrCoeff"=36, "EEPROM_SMBus Address"=46, "EEPROM_ConfigReg"=37] ("Melexis_Cmmds")
        w470 = u8 7 items=["RAM IR raw  Ch1"=4, "RAM IR raw  Ch2"=5, "RAM T_A"=6, "RAM T_OBJ1"=7, "RAM T_OBJ2"=8, "EEPROM_To_max"=32, "EEPROM_To_min"=33, "EEPROM_PWM_CTRL"=34, "EEPROM_Ta_range"=35, "EEPROM_Emissivity_CorrCoeff"=36, "EEPROM_SMBus Address"=46, "EEPROM_ConfigReg"=37] ("Melexis_Cmmds")
        w475 = u8 7 items=["RAM IR raw  Ch1"=4, "RAM IR raw  Ch2"=5, "RAM T_A"=6, "RAM T_OBJ1"=7, "RAM T_OBJ2"=8, "EEPROM_To_max"=32, "EEPROM_To_min"=33, "EEPROM_PWM_CTRL"=34, "EEPROM_Ta_range"=35, "EEPROM_Emissivity_CorrCoeff"=36, "EEPROM_SMBus Address"=46, "EEPROM_ConfigReg"=37] ("Melexis_Cmmds")
        # "Bay 5 Temperature Read"
        # "Bay 4 Temperature Read"
        # "Bay 3 Temperature Read"
        # "Bay 2 Temperature Read"
        # "Bay 1 Temperature Read"
        n272 = local read "Stop Button"() -> (w473:bool)
        n273 = call "IRSensorNIRead.vi"("error in (no error)"=w447, "Melexis_Cmmds"=w475, "Address"=u8 1, "device reference"=w449) -> ("error out"=w446:errorcluster, "Temperature"=w476:dbl, "device reference out"=w472:T2)  [unwired: 5 in]
        n274 = local write "error out"(w446) -> ()
        n275 = Unbundle By Name(w446) -> ("status"=w445:bool)
        n276 = call-poly <vilib>:"PID Control Input Filter.vi"("input"=w476) -> ("output"=w443:dbl)  [unwired: 4 in]
        n277 = case shown="True" w445 {
          tunnel: w443 -> [w485 _]
          tunnel: [w485 w486] -> w444
          frame False {
            n278 = local write "Temperature 1"(w485) -> ()
          }
          frame True {
            n279 = local read "Temperature 1"() -> (w486:dbl)
          }
        }
        n280 = flat-sequence {
          tunnel: w472 -> [w495]
          tunnel: [w495] -> w471
          frame #0 {
            n281 = Wait (ms)(milliseconds to wait=u32 100) -> ()  [unwired: 1 out]
          }
        }
        n282 = call "IRSensorNIRead.vi"("error in (no error)"=w447, "Melexis_Cmmds"=w470, "Address"=u8 2, "device reference"=w471) -> ("error out"=w442:errorcluster, "Temperature"=w468:dbl, "device reference out"=w467:T2)  [unwired: 5 in]
        n283 = Unbundle By Name(w442) -> ("status"=w441:bool)
        n284 = local write "error out"(w442) -> ()
        n285 = call-poly <vilib>:"PID Control Input Filter.vi"("input"=w468) -> ("output"=w440:dbl)  [unwired: 4 in]
        n286 = case shown="True" w441 {
          tunnel: w440 -> [w483 _]
          tunnel: [w483 w484] -> w439
          frame False {
            n287 = local write "Temperature 2"(w483) -> ()
          }
          frame True {
            n288 = local read "Temperature 2"() -> (w484:dbl)
          }
        }
        n289 = flat-sequence {
          tunnel: w467 -> [w493]
          tunnel: [w493] -> w460
          frame #0 {
            n290 = Wait (ms)(milliseconds to wait=u32 100) -> ()  [unwired: 1 out]
          }
        }
        n291 = call "IRSensorNIRead.vi"("error in (no error)"=w447, "Melexis_Cmmds"=w465, "Address"=u8 3, "device reference"=w460) -> ("error out"=w436:errorcluster, "Temperature"=w455:dbl, "device reference out"=w459:T2)  [unwired: 5 in]
        n292 = local write "error out"(w436) -> ()
        n293 = Unbundle By Name(w436) -> ("status"=w435:bool)
        n294 = call-poly <vilib>:"PID Control Input Filter.vi"("input"=w455) -> ("output"=w438:dbl)  [unwired: 4 in]
        n295 = case shown="False" w435 {
          tunnel: w438 -> [w481 _]
          tunnel: [w481 w482] -> w437
          frame False {
            n296 = local write "Temperature 3"(w481) -> ()
          }
          frame True {
            n297 = local read "Temperature 3"() -> (w482:dbl)
          }
        }
        n298 = flat-sequence {
          tunnel: w459 -> [w491]
          tunnel: [w491] -> w457
          frame #0 {
            n299 = Wait (ms)(milliseconds to wait=u32 100) -> ()  [unwired: 1 out]
          }
        }
        n300 = call "IRSensorNIRead.vi"("error in (no error)"=w447, "Melexis_Cmmds"=w466, "Address"=u8 4, "device reference"=w457) -> ("error out"=w431:errorcluster, "Temperature"=w454:dbl, "device reference out"=w458:T2)  [unwired: 5 in]
        n301 = local write "error out"(w431) -> ()
        n302 = Unbundle By Name(w431) -> ("status"=w432:bool)
        n303 = call-poly <vilib>:"PID Control Input Filter.vi"("input"=w454) -> ("output"=w434:dbl)  [unwired: 4 in]
        n304 = case shown="True" w432 {
          tunnel: w434 -> [w479 _]
          tunnel: [w479 w480] -> w433
          frame False {
            n305 = local write "Temperature 4"(w479) -> ()
          }
          frame True {
            n306 = local read "Temperature 4"() -> (w480:dbl)
          }
        }
        n307 = flat-sequence {
          tunnel: w458 -> [w489]
          tunnel: [w489] -> w456
          frame #0 {
            n308 = Wait (ms)(milliseconds to wait=u32 100) -> ()  [unwired: 1 out]
          }
        }
        n309 = call "IRSensorNIRead.vi"("error in (no error)"=w447, "Melexis_Cmmds"=w464, "Address"=u8 5, "device reference"=w456) -> ("error out"=w427:errorcluster, "Temperature"=w453:dbl, "device reference out"=w452:T2)  [unwired: 5 in]
        n310 = flat-sequence {
          tunnel: w452 -> [w487]
          tunnel: [w487] -> w448
          frame #0 {
            n311 = Wait (ms)(milliseconds to wait=u32 100) -> ()  [unwired: 1 out]
          }
        }
        n312 = call-poly <vilib>:"PID Control Input Filter.vi"("input"=w453) -> ("output"=w430:dbl)  [unwired: 4 in]
        n313 = local write "error out"(w427) -> ()
        n314 = Unbundle By Name(w427) -> ("status"=w428:bool)
        n315 = Build Array(w444, w439, w437, w433, w430) -> (w451:dbl[])
        n316 = Array To Cluster(array=w451) -> (cluster=→"Teperature Chart":T1)
        n317 = case shown="False" w428 {
          tunnel: w430 -> [w477 _]
          tunnel: [w477 w478] -> w429
          frame False {
            n318 = local write "Temperature 5"(w477) -> ()
          }
          frame True {
            n319 = local read "Temperature 5"() -> (w478:dbl)
          }
        }
        n320 = script code="MATLAB script"("T1"=w444, "T2"=w439, "T3"=w437, "T4"=w433, "T5"=w429) -> ()  [unwired: 1 in, 1 out]
      }
      n321 = while {
        tunnel: w25 -> [w229]
        stop <- w228 stop-if-true
        n322 = Wait (ms)(milliseconds to wait=u32 400) -> ()  [unwired: 1 out]
        n323 = local read "Temp On? 4"() -> (w227:bool)
        n324 = case shown="True" w227 {
          tunnel: w229 -> [_ w253]
          frame False {
            n325 = local write "Temp SS 4"(TRUE ("Temp SS? 4")) -> ()
          }
          frame True {
            n326 = local read "Set Point 4"() -> (w233:dbl)
            n327 = local read "Temperature 4"() -> (w235:dbl)
            n328 = Subtract(x=w235, y=w233) -> (x-y=w240:dbl)
            n329 = Absolute Value(x=w240) -> (abs(x)=w242:dbl)
            n330 = Less Or Equal?(x=w242, y=1.2) -> (x <= y?=w239:bool)
            n331 = local write "Temp SS 4"(w239) -> ()
            n332 = local read "SSR Duration 4"() -> (w243:dbl)
            n333 = call-poly <vilib>:"PID Online Autotuning.vi"("setpoint"=w233, "manipulated variable"=w243, "autotuning parameters"=T5 {"type of controller"=enum."PID", "relay cycles"=3, "relay amplitude"=1.0, "control specifications"=enum."Normal", "PV noise level"=0.1} ("Autotuning Parameters R1"), "process variable"=w235, "PID gains in"=T4 {"Proportional gain Kc"=0.38538, "Integral time Ti (sec)"=0.524375, "Derivative time Ti (sec)"=0.12585} ("PID gains 2")) -> ("setpoint out"=w245:dbl, "process variable out"=w246:dbl, "PID gains out"=w248:T12)  [unwired: 6 in, 2 out]
            n334 = call <vilib>:"PID Autotuning (Temperature).vi"("desired temperature"=w245, "measured temperature"=w246, "PID gains in"=w248, "output range"=cluster{"output high":dbl, "output low":dbl} {"output high"=3.0, "output low"=-1.0} ("Output range")) -> ("output"=w244:dbl)  [unwired: 12 in, 3 out]
            n335 = Multiply(x=1000.0, y=w244) -> (x*y=w252:dbl)
            n336 = Greater?(x=w233, y=w235) -> (0:w238:bool)
            n337 = Greater Than 0?(x=w252) -> (x > 0?=w236:bool)
            n338 = local write "SSR Duration 4"(w244) -> ()
            n339 = And(x=w236, y=w238) -> (x .and. y?=w237:bool)
            n340 = case shown="True" w237 {
              tunnel: [errorcluster {"status"=FALSE, "code"=0, "source"=""} ("error out") w267] -> _
              tunnel: 5 -> [_ w268]
              tunnel: [w259 w266] -> _
              tunnel: w253 -> [w259 w265]
              tunnel: w252 -> [w258 w264]
              tunnel: [0.0 w263] -> w234
              tunnel: w233 -> [_ w262]
              frame False {
                n341 = Absolute Value(x=w258) -> (abs(x)=w260:dbl)
                n342 = Wait (ms)(milliseconds to wait=w260) -> ()  [unwired: 1 out]
              }
              frame True {
                n343 = call "TurnOnRelayArduino.vi"("channel"=w268, "duration"=w264, "LINX Resource"=w265) -> ("error out"=w267:errorcluster, "LINX Resource Out"=w266:T6)  [unwired: 7 in]
                n344 = script code="tempdiff4= SP4 - T4;\nif tempdiff4 > 10\n  if slope4 < .01\n     temp_check4 = temp_check4 + 1;\n  else\n      temp_check4 =0;\n  end\nend\n\nif temp_check4 > 9\n  temp_error4 = 1\nend"("SP4"=w262) -> ("temp_error4"=w263:dbl)  [unwired: 1 in, 1 out]
              }
            }
            n345 = Not Equal To 0?(x=w234) -> (x != 0?=w232:bool)
            n346 = case shown="True" w232 {
              frame False {
              }
              frame True {
                n347 = local write "Error Message"("Bay 4 Temperature Heating Error") -> ()
              }
            }
            n348 = case shown="True" w232 {
              tunnel: w232 -> [_ w255]
              frame False {
              }
              frame True {
                # "Bay 4 Temperature Controller"
                n349 = local write "Stop Button"(w255) -> ()
              }
            }
          }
        }
        n350 = local read "Stop Button"() -> (w228:bool)
      }
      n351 = while {
        tunnel: w29 -> [w499]
        tunnel: w26 -> [w497]
        stop <- w507 stop-if-true
        # "Pumps"
        n352 = local read "Pump 7"() -> (w498:bool)
        n353 = case shown="True" w498 {
          tunnel: w497 -> [w508 w513]
          frame False {
            n354 = local read "Pump On 7"() -> (w509:bool)
            n355 = case shown="True" w509 {
              tunnel: w508 -> [_ w510]
              frame False {
              }
              frame True {
                n356 = call <instrlib>:"Stop Pump.vi"("VISA resource name"=w510) -> ()  [unwired: 9 in, 2 out]
                n357 = local write "Pump On 7"(FALSE ("Pump On 7")) -> ()
              }
            }
          }
          frame True {
            w515 = u16 0 items=["Infuse", "Withdraw"] ("Run Direction (0:Infuse)")
            w516 = u32 4 items=["milliliters per hour (ml/hr)", "milliliters per minute (ml/min)", "milliliters per second (ml/sec)", "microliters per hour (ul/hr)", "microliters per minute (ul/min)", "microliters per second (ul/sec)", "nanoliters per hour (nl/hr)", "nanoliters per minute (nl/min)", "nanoliters per second (nl/sec)", "picoliters per hour (pl/hr)", "picoliters per minute (pl/min)", "picoliters per second (pl/sec)"] ("Flow Rate Units (1:ml/min)")
            w517 = u16 0 items=["Infuse", "Withdraw"] ("Pump Direction (0:Infuse)")
            n358 = local read "Syringe Pump \n    Flowrate"() -> (w512:dbl)
            n359 = local write "Pump On 7"(TRUE ("Pump On 7")) -> ()
            n360 = call <instrlib>:"Configure Flow Rate & Direction.vi"("VISA resource name"=w513, "Pump Direction (0:Infuse)"=w517, "Flow Rate (5.00)"=w512, "Flow Rate Units (1:ml/min)"=w516) -> ("VISA resource name out"=w514:refnum<visa-resource-name>)  [unwired: 10 in, 1 out]
            n361 = call <instrlib>:"Start Pump.vi"("Run Direction (0:Infuse)"=w515, "VISA resource name"=w514) -> ()  [unwired: 8 in, 2 out]
          }
        }
        n362 = local read "Pump 1"() -> (w506:bool)
        n363 = case shown="True" w506 {
          tunnel: w499 -> [w560 w568]
          frame False {
            n364 = local read "Pump On 1"() -> (w561:bool)
            n365 = case shown="True" w561 {
              tunnel: w560 -> [_ w562]
              frame False {
              }
              frame True {
                n366 = local read "Pump Address 1"() -> (w563:string)
                n367 = local write "Pump On 1"(FALSE ("Pump On 1")) -> ()
                n368 = call "PumpStop.vi"("Pump Address"=w563, "Pump COMM Port"=w562) -> ()  [unwired: 9 in, 1 out]
              }
            }
          }
          frame True {
            n369 = local read "Pump Address 1"() -> (w565:string)
            n370 = local write "Pump On 1"(TRUE ("Pump On 1")) -> ()
            n371 = local read "Flowrate 1"() -> (w566:dbl)
            n372 = call "PumpDispense.vi"("Flowrate(ul/min)"=w566, "Pump Address"=w565, "Pump COMM Port"=w568) -> ()  [unwired: 7 in, 2 out]
          }
        }
        n373 = local read "Stop Button"() -> (w507:bool)
        n374 = Wait (ms)(milliseconds to wait=u32 2000) -> ()  [unwired: 1 out]
        n375 = local read "Pump 2"() -> (w504:bool)
        n376 = case shown="True" w504 {
          tunnel: w499 -> [w551 w559]
          frame False {
            n377 = local read "Pump On 2"() -> (w552:bool)
            n378 = case shown="True" w552 {
              tunnel: w551 -> [_ w553]
              frame False {
              }
              frame True {
                n379 = local read "Pump Address 2"() -> (w554:string)
                n380 = local write "Pump On 2"(FALSE ("Pump On 2")) -> ()
                n381 = call "PumpStop.vi"("Pump Address"=w554, "Pump COMM Port"=w553) -> ()  [unwired: 9 in, 1 out]
              }
            }
          }
          frame True {
            n382 = local read "Pump Address 2"() -> (w556:string)
            n383 = local read "Flowrate 2"() -> (w557:dbl)
            n384 = local write "Pump On 2"(TRUE ("Pump On 2")) -> ()
            n385 = call "PumpDispense.vi"("Flowrate(ul/min)"=w557, "Pump Address"=w556, "Pump COMM Port"=w559) -> ()  [unwired: 7 in, 2 out]
          }
        }
        n386 = local read "Pump 3"() -> (w503:bool)
        n387 = case shown="False" w503 {
          tunnel: w499 -> [w544 w550]
          frame False {
            n388 = local read "Pump On 3"() -> (w543:bool)
            n389 = case shown="True" w543 {
              tunnel: w544 -> [_ w545]
              frame False {
              }
              frame True {
                n390 = local read "Pump Address 3"() -> (w546:string)
                n391 = call "PumpStop.vi"("Pump Address"=w546, "Pump COMM Port"=w545) -> ()  [unwired: 9 in, 1 out]
              }
            }
          }
          frame True {
            n392 = local read "Pump Address 3"() -> (w547:string)
            n393 = local read "Flowrate 3"() -> (w548:dbl)
            n394 = local write "Pump On 3"(TRUE ("Pump On 2")) -> ()
            n395 = call "PumpDispense.vi"("Flowrate(ul/min)"=w548, "Pump Address"=w547, "Pump COMM Port"=w550) -> ()  [unwired: 7 in, 2 out]
          }
        }
        n396 = local read "Pump 4"() -> (w502:bool)
        n397 = case shown="True" w502 {
          tunnel: w499 -> [w536 w542]
          frame False {
            n398 = local read "Pump On 4"() -> (w535:bool)
            n399 = case shown="True" w535 {
              tunnel: w536 -> [_ w537]
              frame False {
              }
              frame True {
                n400 = local read "Pump Address 4"() -> (w538:string)
                n401 = call "PumpStop.vi"("Pump Address"=w538, "Pump COMM Port"=w537) -> ()  [unwired: 9 in, 1 out]
              }
            }
          }
          frame True {
            n402 = local read "Pump Address 4"() -> (w540:string)
            n403 = local read "Flowrate 4"() -> (w541:dbl)
            n404 = local write "Pump On 4"(TRUE ("Pump On 2")) -> ()
            n405 = call "PumpDispense.vi"("Flowrate(ul/min)"=w541, "Pump Address"=w540, "Pump COMM Port"=w542) -> ()  [unwired: 7 in, 2 out]
          }
        }
        n406 = local read "Pump 5"() -> (w501:bool)
        n407 = case shown="False" w501 {
          tunnel: w499 -> [w527 w534]
          frame False {
            n408 = local read "Pump On 5"() -> (w528:bool)
            n409 = case shown="True" w528 {
              tunnel: w527 -> [_ w529]
              frame False {
              }
              frame True {
                n410 = local read "Pump Address 5"() -> (w530:string)
                n411 = call "PumpStop.vi"("Pump Address"=w530, "Pump COMM Port"=w529) -> ()  [unwired: 9 in, 1 out]
              }
            }
          }
          frame True {
            n412 = local read "Pump Address 5"() -> (w531:string)
            n413 = local read "Flowrate 5"() -> (w532:dbl)
            n414 = local write "Pump On 5"(TRUE ("Pump On 2")) -> ()
            n415 = call "PumpDispense.vi"("Flowrate(ul/min)"=w532, "Pump Address"=w531, "Pump COMM Port"=w534) -> ()  [unwired: 7 in, 2 out]
          }
        }
        n416 = local read "Pump 6"() -> (w500:bool)
        n417 = case shown="False" w500 {
          tunnel: w499 -> [w519 w526]
          frame False {
            n418 = local read "Pump On 6"() -> (w520:bool)
            n419 = case shown="True" w520 {
              tunnel: w519 -> [_ w521]
              frame False {
              }
              frame True {
                n420 = local read "Pump Address 6"() -> (w522:string)
                n421 = call "PumpStop.vi"("Pump Address"=w522, "Pump COMM Port"=w521) -> ()  [unwired: 9 in, 1 out]
              }
            }
          }
          frame True {
            n422 = local read "Pump Address 6"() -> (w524:string)
            n423 = local read "Flowrate 6"() -> (w523:dbl)
            n424 = local write "Pump On 6"(TRUE ("Pump On 2")) -> ()
            n425 = call "PumpDispense.vi"("Flowrate(ul/min)"=w523, "Pump Address"=w524, "Pump COMM Port"=w526) -> ()  [unwired: 7 in, 2 out]
          }
        }
      }
      n426 = while {
        tunnel: [w178] -> _
        tunnel: w25 -> [w178]
        stop <- w184 stop-if-true
        n427 = call-poly <vilib>:"Analog Read.vi"("Analog Channel"=u8 0, "LINX Resource"=w178) -> ("Voltage"=w182:dbl)  [unwired: 6 in, 3 out]
        "Phase_Sensor_voltage" <- w182
        n428 = Wait (ms)(milliseconds to wait=u32 300) -> ()  [unwired: 1 out]
        n429 = Build Array(w182) -> (w180:dbl[])
        n430 = Array To Cluster(array=w180) -> (cluster=→"Phase Sensor Chart":T1)
        n431 = local read "Stop Button"() -> (w184:bool)
      }
      n432 = while {
        stop <- w103 stop-if-true
        n433 = script code="TempArr1=circshift(TempArr1,9);\nTempArr2=circshift(TempArr2,9);\nTempArr3=circshift(TempArr3,9);\nTempArr4=circshift(TempArr4,9);\nTempArr5=circshift(TempArr5,9);\n\nTempArr1(10)=T1;\nTempArr2(10)=T2;\nTempArr3(10)=T3;\nTempArr4(10)=T4;\nTempArr5(10)=T5;\n\n[slope1 temp] = polyfit([1,2,3,4,5,6,7,8,9,10]',TempArr1,1);\nslope1 = slope1(1);\n[slope2 temp] = polyfit([1,2,3,4,5,6,7,8,9,10]',TempArr2,1);\nslope2= slope2(1);\n[slope3 temp] = polyfit([1,2,3,4,5,6,7,8,9,10]',TempArr3,1);\nslope3 = slope3(1);\n[slope4 temp] = polyfit([1,2,3,4,5,6,7,8,9,10]',TempArr4,1);\nslope4 = slope4(1);\n[slope5 temp] = polyfit([1,2,3,4,5,6,7,8,9,10]',TempArr5,1);\nslope5 = slope5(1);"() -> ()  [unwired: 1 in, 1 out]
        n434 = Wait (ms)(milliseconds to wait=u32 600) -> ()  [unwired: 1 out]
        n435 = local read "Stop Button"() -> (w103:bool)
      }
    }
    frame #2 {
      w573 = string[] ["e", "f", "g", "h", "i", "j"]
      n436 = local read "COMM Port :: Milligat Pumps"() -> (w572:T3)
      n437 = local read "Error Message"() -> (w575:string)
      n438 = Array Size(array=w573) -> (size(s)=w574:i32)
      n439 = call <instrlib>:"Stop Pump.vi"("VISA resource name"=w570) -> ("error out"=w569:errorcluster)  [unwired: 9 in, 1 out]
      n440 = for {
        N: w574 -> [_]
        tunnel: w573 -> [w577] mode=indexing
        tunnel: w572 -> [w576]
        n441 = call "PumpStop.vi"("Pump Address"=w577, "Pump COMM Port"=w576) -> ()  [unwired: 9 in, 1 out]
      }
      n442 = local write "error out"(w569) -> ()
      n443 = One Button Dialog(message=w575) -> ()  [unwired: 1 in, 1 out]
      n444 = call <vilib>:"Close.vi"("LINX Resource"=w571) -> ()  [unwired: 10 in, 1 out]
    }
  }
